vi "HFRR ADV v08 new software.vi"() -> ()   [LabVIEW 2025] (continued)
        n786 = case shown="True" "LIVE FEED MAX TEMP" {
          selector: "LIVE FEED MAX TEMP" -> [_ w1182]
          frame False {
          }
          frame True {
            n787 = Not(x=w1182) -> (.not. x?=w1181:bool)
            n788 = local write "LIVE FEED MAX TEMP"(w1181) -> ()
            n789 = call "CAMERA LIVE FEED FGV.vi"("Enum - Menu"=CAMERA_LIVE_FEED_ENUM."CAMERA RESTORE") -> ("error out"=w1172:errorcluster)  [unwired: 9 in, 1 out]
            n790 = Type Cast(type=30, x=0) -> (*(type *) &x=w1176:i32)
            n791 = Add(x=w1176, y=48) -> (x+y=w1177:i32)
            n792 = call "CAMERA LIVE FEED FGV.vi"("Enum - Menu"=CAMERA_LIVE_FEED_ENUM."CAMERA MODE SET", "error in (no error)"=w1172, "CAMERA MODE"=w1177) -> ("error out"=w1169:errorcluster)  [unwired: 7 in, 1 out]
            n793 = call "CAMERA LIVE FEED FGV.vi"("Enum - Menu"=CAMERA_LIVE_FEED_ENUM."CAMERA GRAY", "error in (no error)"=w1169) -> ("error out"=w1168:errorcluster)  [unwired: 8 in, 1 out]
            n794 = call "LIST FILE NAMES.vi"("error in (no error)"=w1168) -> ("error out"=w1178:errorcluster, "filenames"=w1179:string[])  [unwired: 9 in]
            n795 = property on="FILE 3" class="CmbBox"(error in=w1178, "Strings[]"=w1179) -> ()  [unwired: 1 in, 2 out]
          }
        }
        n796 = case shown="True" w1161 {
          selector: w1161 -> [_ w1167]
          frame False {
          }
          frame True {
            n797 = Not(x=w1167) -> (.not. x?=w1166:bool)
            n798 = local write "CAMERA ROI MIN TEMP"(w1166) -> ()
            n799 = call "IMAGE ANALYSIS.vi"("Enum"=POST_ANALYSIS_ENUM."MINIMIZE UI") -> ()  [unwired: 9 in, 2 out]
          }
        }
        n800 = local write "CAMERA ROI MAX TEMP"(TRUE ("CAMERA ROI MAX TEMP")) -> ()
        "LIVE FEED MIN TEMP" <- TRUE ("LIVE FEED MIN TEMP")
      }
      frame "Adv Scar Report" {
        n801 = local read "CAMERA ROI MAX TEMP"() -> (w1183:bool)
        n802 = local read "LIVE FEED MIN TEMP"() -> (w1185:bool)
        n803 = local write "LIVE FEED MAX TEMP"(TRUE ("LIVE FEED MAX TEMP")) -> ()
        n804 = case shown="True" w1185 {
          selector: w1185 -> [_ w1194]
          frame False {
          }
          frame True {
            n805 = Not(x=w1194) -> (.not. x?=w1193:bool)
            n806 = local write "LIVE FEED MIN TEMP"(w1193) -> ()
            n807 = call "CAMERA LIVE FEED FGV.vi"("Enum - Menu"=CAMERA_LIVE_FEED_ENUM."CAMERA MINIMIZE") -> ()  [unwired: 9 in, 2 out]
          }
        }
        n808 = case shown="True" w1183 {
          selector: w1183 -> [_ w1191]
          frame False {
          }
          frame True {
            n809 = Not(x=w1191) -> (.not. x?=w1189:bool)
            n810 = local write "CAMERA ROI MAX TEMP"(w1189) -> ()
            n811 = call "IMAGE ANALYSIS.vi"("Enum"=POST_ANALYSIS_ENUM."SHOW UI") -> ("error out"=w1188:errorcluster)  [unwired: 9 in, 1 out]
            n812 = call "LIST FILE NAMES.vi"("error in (no error)"=w1188) -> ("filenames"=w1187:string[])  [unwired: 9 in, 1 out]
            n813 = property on="Test File List :" class="CmbBox"("Strings[]"=w1187) -> ()  [unwired: 2 in, 2 out]
          }
        }
        n814 = local write "CAMERA ROI MIN TEMP"(TRUE ("CAMERA ROI MIN TEMP")) -> ()
      }
      frame "Compare Files" {
        n815 = local read "LIVE FEED MIN TEMP"() -> (w1197:bool)
        n816 = local write "LIVE FEED MAX TEMP"(TRUE ("LIVE FEED MAX TEMP")) -> ()
        n817 = local read "CAMERA ROI MIN TEMP"() -> (w1195:bool)
        n818 = case shown="True" w1197 {
          selector: w1197 -> [_ w1204]
          frame False {
          }
          frame True {
            n819 = Not(x=w1204) -> (.not. x?=w1203:bool)
            n820 = local write "LIVE FEED MIN TEMP"(w1203) -> ()
            n821 = call "CAMERA LIVE FEED FGV.vi"("Enum - Menu"=CAMERA_LIVE_FEED_ENUM."CAMERA MINIMIZE") -> ()  [unwired: 9 in, 2 out]
          }
        }
        n822 = case shown="True" w1195 {
          selector: w1195 -> [_ w1201]
          frame False {
          }
          frame True {
            n823 = Not(x=w1201) -> (.not. x?=w1200:bool)
            n824 = local write "CAMERA ROI MIN TEMP"(w1200) -> ()
            n825 = call "IMAGE ANALYSIS.vi"("Enum"=POST_ANALYSIS_ENUM."MINIMIZE UI") -> ()  [unwired: 9 in, 2 out]
          }
        }
        n826 = local write "CAMERA ROI MAX TEMP"(TRUE ("CAMERA ROI MAX TEMP")) -> ()
      }
      frame "About" {
        n827 = local read "LIVE FEED MIN TEMP"() -> (w1207:bool)
        n828 = local write "LIVE FEED MAX TEMP"(TRUE ("LIVE FEED MAX TEMP")) -> ()
        n829 = local read "CAMERA ROI MIN TEMP"() -> (w1206:bool)
        n830 = case shown="True" w1207 {
          selector: w1207 -> [_ w1214]
          frame False {
          }
          frame True {
            n831 = Not(x=w1214) -> (.not. x?=w1213:bool)
            n832 = local write "LIVE FEED MIN TEMP"(w1213) -> ()
            n833 = call "CAMERA LIVE FEED FGV.vi"("Enum - Menu"=CAMERA_LIVE_FEED_ENUM."CAMERA MINIMIZE") -> ()  [unwired: 9 in, 2 out]
          }
        }
        n834 = case shown="True" w1206 {
          selector: w1206 -> [_ w1211]
          frame False {
          }
          frame True {
            n835 = Not(x=w1211) -> (.not. x?=w1210:bool)
            n836 = local write "CAMERA ROI MIN TEMP"(w1210) -> ()
            n837 = call "IMAGE ANALYSIS.vi"("Enum"=POST_ANALYSIS_ENUM."MINIMIZE UI") -> ()  [unwired: 9 in, 2 out]
          }
        }
        n838 = local write "CAMERA ROI MAX TEMP"(TRUE ("CAMERA ROI MIN TEMP")) -> ()
      }
      frame "Advance" {
        n839 = local read "LIVE FEED MIN TEMP"() -> (w1217:bool)
        n840 = local write "LIVE FEED MAX TEMP"(TRUE ("LIVE FEED MAX TEMP")) -> ()
        n841 = local read "CAMERA ROI MIN TEMP"() -> (w1215:bool)
        n842 = case shown="True" w1217 {
          selector: w1217 -> [_ w1224]
          frame False {
          }
          frame True {
            n843 = Not(x=w1224) -> (.not. x?=w1223:bool)
            n844 = local write "LIVE FEED MIN TEMP"(w1223) -> ()
            n845 = call "CAMERA LIVE FEED FGV.vi"("Enum - Menu"=CAMERA_LIVE_FEED_ENUM."CAMERA MINIMIZE") -> ()  [unwired: 9 in, 2 out]
          }
        }
        n846 = local write "CAMERA ROI MAX TEMP"(TRUE ("CAMERA ROI MAX TEMP")) -> ()
        n847 = case shown="True" w1215 {
          selector: w1215 -> [_ w1221]
          frame False {
          }
          frame True {
            n848 = Not(x=w1221) -> (.not. x?=w1220:bool)
            n849 = local write "CAMERA ROI MIN TEMP"(w1220) -> ()
            n850 = call "IMAGE ANALYSIS.vi"("Enum"=POST_ANALYSIS_ENUM."MINIMIZE UI") -> ()  [unwired: 9 in, 2 out]
          }
        }
      }
      frame "Mooha" {
        n851 = local read "LIVE FEED MIN TEMP"() -> (w1227:bool)
        n852 = local write "LIVE FEED MAX TEMP"(TRUE ("LIVE FEED MAX TEMP")) -> ()
        n853 = local read "CAMERA ROI MIN TEMP"() -> (w1225:bool)
        n854 = case shown="True" w1227 {
          selector: w1227 -> [_ w1234]
          frame False {
          }
          frame True {
            n855 = Not(x=w1234) -> (.not. x?=w1233:bool)
            n856 = local write "LIVE FEED MIN TEMP"(w1233) -> ()
            n857 = call "CAMERA LIVE FEED FGV.vi"("Enum - Menu"=CAMERA_LIVE_FEED_ENUM."CAMERA MINIMIZE") -> ()  [unwired: 9 in, 2 out]
          }
        }
        n858 = local write "CAMERA ROI MAX TEMP"(TRUE ("CAMERA ROI MAX TEMP")) -> ()
        n859 = case shown="True" w1225 {
          selector: w1225 -> [_ w1231]
          frame False {
          }
          frame True {
            n860 = Not(x=w1231) -> (.not. x?=w1230:bool)
            n861 = local write "CAMERA ROI MIN TEMP"(w1230) -> ()
            n862 = call "IMAGE ANALYSIS.vi"("Enum"=POST_ANALYSIS_ENUM."MINIMIZE UI") -> ()  [unwired: 9 in, 2 out]
          }
        }
      }
    }
    n863 = local read "Auto Start Test"() -> (w971:bool)
    n864 = case shown="True" "sign in temp" {
      frame False {
      }
      frame True {
        w1007 = 1 ("y")
        n865 = local read "USERNAME"() -> (w1013:string)
        n866 = local read "USER ID"() -> (w1010:string)
        n867 = call <vilib>:"Trim Whitespace.vi"("string"=w1013) -> ("trimmed string"=w1012:string)  [unwired: 1 in]
        n868 = call <vilib>:"Trim Whitespace.vi"("string"=w1010) -> ("trimmed string"=w1011:string)  [unwired: 1 in]
        n869 = String Length(string=w1012) -> (length=w1009:i32)
        n870 = String Length(string=w1011) -> (length=w1008:i32)
        n871 = Greater?(x=w1009, y=w1007) -> (0:w1006:bool)
        n872 = Greater?(x=w1008, y=w1007) -> (0:w1005:bool)
        n873 = And(x=w1006, y=w1005) -> (x .and. y?=w1004:bool)
        n874 = case shown="True" w1004 {
          frame False {
            n875 = property on="Sign In" class="Bool (strict)"("DisabledEnum"=T16."Disabled" ("Disabled")) -> ()  [unwired: 2 in, 2 out]
          }
          frame True {
            n876 = property on="Sign In" class="Bool (strict)"("DisabledEnum"=T16."Enabled" ("Disabled")) -> ()  [unwired: 2 in, 2 out]
          }
        }
      }
    }
    n877 = local read "Air Temperature"() -> (w988:bool)
    n878 = local read "Coefficient Of Friction"() -> (w989:bool)
    n879 = case shown="False" w971 {
      frame False {
        n880 = local read "Auto stop temp"() -> (w1001:bool)
        n881 = case shown="True" w1001 {
          frame False {
          }
          frame True {
            n882 = local write "Auto Start Temp"(FALSE ("Auto Start Temp")) -> ()
          }
        }
      }
      frame True {
        "Auto stop temp" <- TRUE ("Auto stop temp")
      }
    }
    n883 = local read "Humidity"() -> (w987:bool)
    n884 = case shown="\"HOME\"" w998 {
      frame "HOME" {
        n885 = local write "main tab sub"(enum32{"Page 1", "Page 2"}."Page 1" ("main tab sub")) -> ()
      }
      frame Default {
        n886 = local write "main tab sub"(enum32{"Page 1", "Page 2"}."Page 2" ("main tab sub")) -> ()
      }
    }
    n887 = case shown="True" w997 {
      selector: w997 -> [_ w1340]
      frame False {
      }
      frame True {
        n888 = Not(x=w1340) -> (.not. x?=w1339:bool)
        n889 = local write "Sign In"(w1339) -> ()
        n890 = local write "Main Dashboard Buttons"(T22."Test Setup" ("Main Dashboard Buttons")) -> ()
      }
    }
    n891 = case shown="\"Numeric Display\", Default" "Num/Graph" {
      frame "Numeric Display", Default {
        n892 = property on="Single/Multiple" class="RadioBtnsControl (strict)"("Visible"=FALSE) -> ()  [unwired: 2 in, 2 out]
        n893 = property on="Single - Graph" class="Ring (strict)"("Visible"=FALSE) -> ()  [unwired: 2 in, 2 out]
        n894 = local write "Main Tab Display"(T4."Dashboard 1" ("Main Tab Display")) -> ()
      }
      frame "Graph Display" {
        n895 = property on="Single/Multiple" class="RadioBtnsControl (strict)"("Visible"=TRUE) -> ()  [unwired: 2 in, 2 out]
        n896 = case shown="\"Multiple\"" "Single/Multiple" {
          frame "Single ", Default {
            n897 = property on="Single - Graph" class="Ring (strict)"("Visible"=TRUE) -> ()  [unwired: 2 in, 2 out]
            n898 = local write "Main Tab Display"(T4."Dashboard 3" ("Main Tab Display")) -> ()
          }
          frame "Multiple" {
            n899 = property on="Single - Graph" class="Ring (strict)"("Visible"=FALSE) -> ()  [unwired: 2 in, 2 out]
            n900 = local write "Main Tab Display"(T4."Dashboard 2" ("Main Tab Display")) -> ()
          }
        }
      }
    }
    n901 = local read "Stroke"() -> (w986:bool)
    n902 = local read "USERNAME"() -> (w992:string)
    n903 = local read "USER ID"() -> (w991:string)
    n904 = case shown="True" w989 {
      selector: w989 -> [_ w1274]
      frame False {
      }
      frame True {
        n905 = Not(x=w1274) -> (.not. x?=w1273:bool)
        n906 = local write "Coefficient Of Friction"(w1273) -> ()
        n907 = local write "Tab Control 2"(T6."Coefficient Of Friction" ("Tab Control 2")) -> ()
      }
    }
    n908 = case shown="True" w988 {
      selector: w988 -> [_ w1271]
      frame False {
      }
      frame True {
        n909 = Not(x=w1271) -> (.not. x?=w1269:bool)
        n910 = local write "Air Temperature"(w1269) -> ()
        n911 = local write "Tab Control 2"(T6."Air Temperature" ("Tab Control 2")) -> ()
      }
    }
    n912 = local write "Operator ID"(w991) -> ()
    n913 = case shown="True" w986 {
      selector: w986 -> [_ w1265]
      frame False {
      }
      frame True {
        n914 = Not(x=w1265) -> (.not. x?=w1263:bool)
        n915 = local write "Stroke"(w1263) -> ()
        n916 = local write "Tab Control 2"(T6."Stroke" ("Tab Control 2")) -> ()
      }
    }
    n917 = local write "tested by"(w992) -> ()
    n918 = case shown="True" w987 {
      selector: w987 -> [_ w1268]
      frame False {
      }
      frame True {
        n919 = Not(x=w1268) -> (.not. x?=w1266:bool)
        n920 = local write "Humidity"(w1266) -> ()
        n921 = local write "Tab Control 2"(T6."Humidity" ("Tab Control 2")) -> ()
      }
    }
    n922 = case shown="\"Calibration\"" "Main Dashboard Buttons" {
      tunnel: [T2."HOME" ("Main Tab") T2."Test Setup" ("Main Tab") T2."Acquire" ("Main Tab") T2."Adv Scar" ("Main Tab") T2."Adv Scar Report" ("Main Tab") T2."Compare Files" ("Main Tab") T2."Calibration" ("Main Tab") T2."About" ("Main Tab") T2."Advance" ("Main Tab")] -> w970
      frame "Home", Default {
      }
      frame "Test Setup" {
      }
      frame "Dashboard" {
      }
      frame "Imaging" {
      }
      frame "Report" {
      }
      frame "Analysis" {
      }
      frame "Calibration" {
      }
      frame "About" {
      }
      frame "Advance" {
      }
    }
    n923 = Wait (ms)(milliseconds to wait=u32 100) -> ()  [unwired: 1 out]
    n924 = local read "Main Tab Display"() -> (w990:T4)
    n925 = local write "Main Tab"(w970) -> ()
    n926 = case shown="\"Dashboard 3\"" w990 {
      frame "Dashboard 1", Default {
        n927 = property on="Reset Graph" class="Bool (strict)"("Visible"=FALSE) -> ()  [unwired: 2 in, 2 out]
      }
      frame "Dashboard 2" {
        n928 = property on="Reset Graph" class="Bool (strict)"("Visible"=TRUE) -> ()  [unwired: 2 in, 2 out]
      }
      frame "Dashboard 3" {
        n929 = property on="Reset Graph" class="Bool (strict)"("Visible"=TRUE) -> ()  [unwired: 2 in, 2 out]
      }
    }
    n930 = local read "SCAR MEASURMENT"() -> (w978:enum32{"Auto Scar", "Manual Scar"})
    n931 = local read "Humidity"() -> (w993:bool)
    n932 = local read "Cap Live Image"() -> (w975:bool)
    n933 = local read "Sample Temperature"() -> (w985:bool)
    n934 = local read "Air Temp vs Humidity"() -> (w983:bool)
    n935 = local read "Frequency"() -> (w984:bool)
    n936 = case shown="False" w993 {
      frame False {
        n937 = local write "Humidity On Command"(TRUE ("Humidity On Command")) -> ()
        n938 = case shown="True" "Humidity Off Command" {
          selector: "Humidity Off Command" -> [_ w1281]
          frame False {
          }
          frame True {
            n939 = stacked-sequence {
              frame #0 {
                n940 = local read "WriteHumidity"() -> (w1283:string[])
                n941 = Insert Into Array(array=w1283, new element="R;1" ("new element/subarray")) -> (w1284:string[])  [unwired: 1 in]
                n942 = local write "WriteHumidity"(w1284) -> ()
              }
              frame #1 {
                n943 = Wait (ms)(milliseconds to wait=u32 2000) -> ()  [unwired: 1 out]
              }
              frame #2 {
                n944 = local read "EVENT LOG"() -> (w1290:string)
                n945 = local read "WriteHumidity"() -> (w1287:string[])
                n946 = call "Event Log.vi"("Content"="Humidity Control Off" ("string"), "EVENT LOG"=w1290) -> ("EVENT LOG"=w1291:string)  [unwired: 8 in, 1 out]
                n947 = local write "EVENT LOG"(w1291) -> ()
                n948 = Insert Into Array(array=w1287, new element="R;1" ("new element/subarray")) -> (w1288:string[])  [unwired: 1 in]
                n949 = local write "WriteHumidity"(w1288) -> ()
              }
            }
            n950 = Not(x=w1281) -> (.not. x?=w1280:bool)
            n951 = local write "Humidity Off Command"(w1280) -> ()
          }
        }
      }
      frame True {
        n952 = local write "Humidity Off Command"(TRUE ("Humidity Off Command")) -> ()
        n953 = case shown="False" "Humidity On Command" {
          selector: "Humidity On Command" -> [_ w1295]
          frame False {
          }
          frame True {
            n954 = stacked-sequence {
              frame #0 {
                n955 = local read "Set Rh"() -> (w1301:dbl)
                n956 = Number To Fractional String(number=w1301, precision (6)=i16 2) -> (F-format string=w1302:string)  [unwired: 2 in]
                n957 = local read "WriteHumidity"() -> (w1299:string[])
                n958 = Concatenate Strings("M;" ("new element/subarray"), w1302) -> (w1300:string)
                n959 = Insert Into Array(array=w1299, new element=w1300) -> (w1298:string[])  [unwired: 1 in]
                n960 = local write "WriteHumidity"(w1298) -> ()
              }
              frame #1 {
                n961 = Wait (ms)(milliseconds to wait=u32 1500) -> ()  [unwired: 1 out]
              }
              frame #2 {
                (unwired) "% RH" ("string")
                (unwired) i16 2 ("precision (6)")
                (unwired) "M;" ("new element/subarray")
                n962 = local read "Set Rh"() -> (w1309:dbl)
                n963 = Number To Fractional String(number=w1309, precision (6)=i16 2) -> (F-format string=w1306:string)  [unwired: 2 in]
                n964 = local read "WriteHumidity"() -> (w1311:string[])
                n965 = Concatenate Strings("M;" ("new element/subarray"), w1306) -> (w1310:string)
                n966 = Concatenate Strings("Humidity Set to : " ("string"), w1306, "% RH" ("string")) -> (w1304:string)
                n967 = Insert Into Array(array=w1311, new element=w1310) -> (w1312:string[])  [unwired: 1 in]
                n968 = disable-structure shown="Enabled" {
                  frame Enabled {
                    n969 = local read "EVENT LOG"() -> (w1315:string)
                    n970 = call "Event Log.vi"("Content"="Humidity Control On", "EVENT LOG"=w1315) -> ("EVENT LOG"=w1316:string)  [unwired: 8 in, 1 out]
                    n971 = local write "EVENT LOG"(w1316) -> ()
                  }
                  frame Disabled {
                  }
                }
                n972 = disable-structure shown="Enabled" {
                  disable-tunnel: w1304 -> [_ _]
                  frame Enabled {
                    n973 = local read "EVENT LOG"() -> (w1318:string)
                    n974 = call "Event Log.vi"("Content"="Humidity Control On", "EVENT LOG"=w1318) -> ("EVENT LOG"=w1319:string)  [unwired: 8 in, 1 out]
                    n975 = local write "EVENT LOG"(w1319) -> ()
                  }
                  frame Disabled {
                  }
                }
                n976 = local write "WriteHumidity"(w1312) -> ()
              }
            }
            n977 = Not(x=w1295) -> (.not. x?=w1294:bool)
            n978 = local write "Humidity On Command"(w1294) -> ()
          }
        }
      }
    }
    n979 = Equal?(x=w978, y=enum32{"Auto Scar", "Manual Scar"}."Auto Scar" ("SCAR MEASURMENT")) -> (x = y?=w974:bool)
    n980 = local read "TEST STANDARD"() -> (w981:T3)
    n981 = And(x=w975, y=w974) -> (x .and. y?=w976:bool)
    n982 = case shown="True" w976 {
      selector: w976 -> [_ w1080]
      tunnel: errorcluster {"status"=FALSE, "code"=0, "source"=""} ("error in (no error) 3") -> [_ w1081]
      frame False {
      }
      frame True {
        n983 = stacked-sequence {
          tunnel: w1081 -> [_ _ _ _ _ _ _ w1129]
          tunnel: w1080 -> [_ _ _ _ _ w1110 _ _]
          frame #0 {
            n984 = call "CAMERA LIVE FEED FGV.vi"("Enum - Menu"=CAMERA_LIVE_FEED_ENUM."CAMERA MINIMIZE") -> ()  [unwired: 9 in, 2 out]
          }
          frame #1 {
            n985 = property on="Auto Scar Check  2" class="Clust (strict)"("Visible"=TRUE) -> ()  [unwired: 2 in, 2 out]
          }
          frame #2 {
            n986 = String To Path(string="C:\\LAB-IQ\\Image Calibrate v01.dcf") -> (path=w1086:path)
            n987 = Open/Create/Replace File ("Open File")(file path (use dialog)=w1086) -> (refnum out=w1087:refnum<file>)  [unwired: 5 in, 2 out]
            n988 = for {
              N: 4 -> [_]
              tunnel: w1087 -> [w1093]
              i -> [w1089]
              n989 = Read from Text File ("Read File")(file (use dialog)=w1093) -> (text=w1094:string)  [unwired: 3 in, 3 out]
              n990 = String Subset(string=w1094, offset (0)=6, length (rest)=10 ("length (rest)")) -> (substring=w1090:string)
              n991 = Fract/Exp String To Number(string=w1090) -> (number=w1088:dbl)  [unwired: 3 in, 1 out]
              n992 = case shown="0" w1089 {
                tunnel: w1088 -> [w1095 w1096 _ w1097 _]
                frame 0 {
                  "5x Gain" <- w1095
                }
                frame 1 {
                  "10x Gain" <- w1096
                }
                frame 2 {
                }
                frame 3 {
                  "100x gain" <- w1097
                }
                frame 4, Default {
                }
              }
            }
          }
          frame #3 {
            n993 = local read "FILE 3"() -> (w1103:string)
            n994 = call <vilib>:"Trim Whitespace.vi"("string"="C:\\LAB-IQ\\images\\") -> ("trimmed string"=w1105:string)  [unwired: 1 in]
            n995 = String To Path(string=w1105) -> (path=w1104:path)
            n996 = Concatenate Strings(w1103, ".png" ("string")) -> (w1102:string)
            n997 = Build Path(base path=w1104, name or relative path=w1102) -> (appended path=w1100:path)
            "Image path" <- w1100
            n998 = Path To String(path=w1100) -> (string=w1099:string)
            n999 = call "CAMERA LIVE FEED FGV.vi"("Enum - Menu"=CAMERA_LIVE_FEED_ENUM."CAMERA SAVE", "Image Path"=w1099) -> ()  [unwired: 8 in, 2 out]
          }
          frame #4 {
            n1000 = One Button Dialog(message="Image saved successfully") -> ()  [unwired: 1 in, 1 out]
          }
          frame #5 {
            n1001 = local read "TEST STANDARD"() -> (w1109:T3)
            n1002 = local read "Magnification len live scar"() -> (w1121:string)
            n1003 = Not(x=w1110) -> (.not. x?=w1111:bool)
            n1004 = local write "Cap Live Image"(w1111) -> ()
            n1005 = case shown="\"ISO 12156\"" w1109 {
              tunnel: ["ASTM D6079" "ISO 12156"] -> w1108
              frame "ASTM D6079", Default {
              }
              frame "ISO 12156" {
              }
            }
            n1006 = case shown="\"5x\", Default" w1121 {
              tunnel: [w1124 w1125] -> w1120
              frame "5x", Default {
                n1007 = local read "5x Gain"() -> (w1124:dbl)
              }
              frame "10x" {
                # "5x"
                n1008 = local read "10x Gain"() -> (w1125:dbl)
              }
            }
            n1009 = local read "Image path"() -> (w1119:path)
            n1010 = local read "FILE 3"() -> (w1112:string)
            n1011 = call "EDGE DETCTION.vi"("GAIN VALUE"=w1120, "Image Path"=w1119) -> ("error out"=w1118:errorcluster, "return value"=w1117:cluster{string, string, dbl, dbl, dbl})  [unwired: 8 in]
            n1012 = Bundle By Name(cluster=T23 {"File Name"="", "Test Method"="", "Operator"="", "Fuel Description"="", "Date and time"=""} ("Main Ref"), "File Name"=w1112, "Test Method"=w1108) -> (w1113:T23)
            n1013 = call "duf file read.vi"("error in (no error)"=w1118, "Main Ref"=w1113) -> ("error out"=w1116:errorcluster, "Main Ref 2"=w1114:T23)  [unwired: 8 in]
            n1014 = call "EDGE DETECTION REPORT.vi"("error in (no error)"=w1116, "return value 2"=w1117, "Main Ref"=w1114) -> ()  [unwired: 8 in, 1 out]
          }
          frame #6 {
            n1015 = property on="Auto Scar Check  2" class="Clust (strict)"("Visible"=FALSE) -> ()  [unwired: 2 in, 2 out]
          }
          frame #7 {
            n1016 = call "CAMERA LIVE FEED FGV.vi"("Enum - Menu"=CAMERA_LIVE_FEED_ENUM."CAMERA MINIMIZE", "error in (no error)"=w1129) -> ()  [unwired: 8 in, 2 out]
            n1017 = local write "Main Dashboard Buttons"(T1."Home" ("Main Dashboard Buttons")) -> ()
            n1018 = local write "Main Tab"(T2."HOME" ("Main Tab")) -> ()
          }
        }
      }
    }
    n1019 = local read "Heater Button"() -> (w982:bool)
    n1020 = case shown="True" w984 {
      selector: w984 -> [_ w1259]
      frame False {
      }
      frame True {
        n1021 = Not(x=w1259) -> (.not. x?=w1257:bool)
        n1022 = local write "Frequency"(w1257) -> ()
        n1023 = local write "Tab Control 2"(T6."Frequency" ("Tab Control 2")) -> ()
      }
    }
    n1024 = case shown="True" w983 {
      selector: w983 -> [_ w1256]
      frame False {
      }
      frame True {
        n1025 = Not(x=w1256) -> (.not. x?=w1254:bool)
        n1026 = local write "Air Temp vs Humidity"(w1254) -> ()
        n1027 = local write "Tab Control 2"(T6."Air Temp vs Rh" ("Tab Control 2")) -> ()
      }
    }
    n1028 = case shown="True" w985 {
      selector: w985 -> [_ w1262]
      frame False {
      }
      frame True {
        n1029 = Not(x=w1262) -> (.not. x?=w1260:bool)
        n1030 = local write "Sample Temperature"(w1260) -> ()
        n1031 = local write "Tab Control 2"(T6."Sample Temperature" ("Tab Control 2")) -> ()
      }
    }
    n1032 = case shown="\"Custom\"" w981 {
      frame "ASTM D6079", Default {
        w1235 = "ASTM D6079 TEST CONDITIONS" ("Standard 2")
        n1033 = local write "Standard 2"(w1235) -> ()
        n1034 = local write "Standard"(w1235) -> ()
      }
      frame "ISO 12156" {
        w1236 = "ISO 12156 TEST CONDITIONS" ("Standard 2")
        n1035 = local write "Standard 2"(w1236) -> ()
        n1036 = local write "Standard"(w1236) -> ()
      }
      frame "CEC F-096-A-06" {
        w1237 = "CEC F-096-A-06 TEST CONDITIONS" ("Standard 2")
        n1037 = local write "Standard 2"(w1237) -> ()
        n1038 = local write "Standard"(w1237) -> ()
      }
      frame "Custom" {
        w1238 = "CUSTOM TEST CONDITIONS" ("Standard 2")
        n1039 = local write "Standard 2"(w1238) -> ()
        n1040 = local write "Standard"(w1238) -> ()
      }
    }
    n1041 = case shown="True" w982 {
      frame False {
        n1042 = local write "Temperature On Command"(TRUE ("Temperature On Command")) -> ()
        n1043 = case shown="True" "Temperature Off Command" {
          selector: "Temperature Off Command" -> [_ w1242]
          frame False {
          }
          frame True {
            n1044 = Not(x=w1242) -> (.not. x?=w1241:bool)
            n1045 = local read "EVENT LOG"() -> (w1245:string)
            n1046 = local write "Temperature Off Command"(w1241) -> ()
            n1047 = call "Event Log.vi"("Content"="Heater Off", "EVENT LOG"=w1245) -> ("EVENT LOG"=w1244:string)  [unwired: 8 in, 1 out]
            n1048 = local write "EVENT LOG"(w1244) -> ()
          }
        }
      }
      frame True {
        n1049 = local write "Temperature Off Command"(TRUE ("Temperature Off Command")) -> ()
        n1050 = case shown="True" "Temperature On Command" {
          selector: "Temperature On Command" -> [_ w1249]
          frame False {
          }
          frame True {
            n1051 = Not(x=w1249) -> (.not. x?=w1248:bool)
            n1052 = local write "Temperature On Command"(w1248) -> ()
            n1053 = disable-structure shown="Enabled" {
              disable-tunnel: "Heater On" -> [w1251 _]
              frame Enabled {
                n1054 = local read "EVENT LOG"() -> (w1252:string)
                n1055 = call "Event Log.vi"("Content"=w1251, "EVENT LOG"=w1252) -> ("EVENT LOG"=w1253:string)  [unwired: 8 in, 1 out]
                n1056 = local write "EVENT LOG"(w1253) -> ()
              }
              frame Disabled {
              }
            }
          }
        }
      }
    }
    n1057 = local read "Main Tab"() -> (w973:T2)
    n1058 = case shown="\"About\"" w973 {
      frame "HOME", Default {
        w1016 = T16."Enabled" ("Disabled")
        n1059 = local read "Service Password enable"() -> (w1018:bool)
        n1060 = property on="Imaging" class="Bool (strict)"("DisabledEnum"=w1016) -> ()  [unwired: 2 in, 2 out]
        n1061 = property on="Dashboard" class="Bool (strict)"("DisabledEnum"=w1016) -> ()  [unwired: 2 in, 2 out]
        n1062 = property on="Test Setup" class="Bool (strict)"("DisabledEnum"=w1016) -> ()  [unwired: 2 in, 2 out]
        n1063 = property on="Analysis" class="Bool (strict)"("DisabledEnum"=w1016) -> ()  [unwired: 2 in, 2 out]
        n1064 = property on="Home" class="Bool (strict)"("DisabledEnum"=w1016) -> ()  [unwired: 2 in, 2 out]
        n1065 = property on="Report" class="Bool (strict)"("DisabledEnum"=w1016) -> ()  [unwired: 2 in, 2 out]
        n1066 = property on="Main Dashboard Buttons" class="RadioBtnsControl (strict)"("DisabledEnum"=w1016) -> ()  [unwired: 2 in, 2 out]
        n1067 = property on="Calibration" class="Bool (strict)"("DisabledEnum"=w1016) -> ()  [unwired: 2 in, 2 out]
        n1068 = case shown="True" w1018 {
          tunnel: [T16."Disabled" ("Disabled") T16."Enabled" ("Disabled")] -> w1017
          frame False {
          }
          frame True {
          }
        }
        n1069 = property on="About" class="Bool (strict)"("DisabledEnum"=w1017) -> ()  [unwired: 2 in, 2 out]
      }
      frame "Test Setup" {
        w1023 = T16."Enabled" ("Disabled")
        n1070 = local read "Service Password enable"() -> (w1022:bool)
        n1071 = property on="Dashboard" class="Bool (strict)"("DisabledEnum"=T16."Disabled" ("Disabled")) -> ()  [unwired: 2 in, 2 out]
        n1072 = property on="Imaging" class="Bool (strict)"("DisabledEnum"=w1023) -> ()  [unwired: 2 in, 2 out]
        n1073 = property on="Analysis" class="Bool (strict)"("DisabledEnum"=w1023) -> ()  [unwired: 2 in, 2 out]
        n1074 = property on="Home" class="Bool (strict)"("DisabledEnum"=w1023) -> ()  [unwired: 2 in, 2 out]
        n1075 = property on="Report" class="Bool (strict)"("DisabledEnum"=w1023) -> ()  [unwired: 2 in, 2 out]
        n1076 = property on="Test Setup" class="Bool (strict)"("DisabledEnum"=w1023) -> ()  [unwired: 2 in, 2 out]
        n1077 = case shown="True" w1022 {
          tunnel: [T16."Disabled" ("Disabled") T16."Enabled" ("Disabled")] -> w1021
          frame False {
          }
          frame True {
          }
        }
        n1078 = property on="About" class="Bool (strict)"("DisabledEnum"=w1021) -> ()  [unwired: 2 in, 2 out]
      }
      frame "Adv Scar" {
        w1030 = T16."Enabled" ("Disabled")
        n1079 = property on="Dashboard" class="Bool (strict)"("DisabledEnum"=T16."Disabled" ("Disabled")) -> ()  [unwired: 2 in, 2 out]
        n1080 = property on="Imaging" class="Bool (strict)"("DisabledEnum"=w1030) -> ()  [unwired: 2 in, 2 out]
        n1081 = property on="Analysis" class="Bool (strict)"("DisabledEnum"=w1030) -> ()  [unwired: 2 in, 2 out]
        n1082 = property on="Home" class="Bool (strict)"("DisabledEnum"=w1030) -> ()  [unwired: 2 in, 2 out]
        n1083 = property on="Report" class="Bool (strict)"("DisabledEnum"=w1030) -> ()  [unwired: 2 in, 2 out]
        n1084 = property on="Test Setup" class="Bool (strict)"("DisabledEnum"=w1030) -> ()  [unwired: 2 in, 2 out]
        n1085 = local read "Service Password enable"() -> (w1028:bool)
        n1086 = case shown="True" w1028 {
          tunnel: [T16."Disabled" ("Disabled") T16."Enabled" ("Disabled")] -> w1027
          frame False {
          }
          frame True {
          }
        }
        n1087 = property on="About" class="Bool (strict)"("DisabledEnum"=w1027) -> ()  [unwired: 2 in, 2 out]
      }
      frame "Calibration" {
        w1033 = T16."Enabled" ("Disabled")
        n1088 = property on="Dashboard" class="Bool (strict)"("DisabledEnum"=T16."Disabled" ("Disabled")) -> ()  [unwired: 2 in, 2 out]
        n1089 = property on="Imaging" class="Bool (strict)"("DisabledEnum"=w1033) -> ()  [unwired: 2 in, 2 out]
        n1090 = property on="Analysis" class="Bool (strict)"("DisabledEnum"=w1033) -> ()  [unwired: 2 in, 2 out]
        n1091 = property on="Home" class="Bool (strict)"("DisabledEnum"=w1033) -> ()  [unwired: 2 in, 2 out]
        n1092 = property on="Report" class="Bool (strict)"("DisabledEnum"=w1033) -> ()  [unwired: 2 in, 2 out]
        n1093 = property on="Test Setup" class="Bool (strict)"("DisabledEnum"=w1033) -> ()  [unwired: 2 in, 2 out]
        n1094 = local read "Service Password enable"() -> (w1035:bool)
        n1095 = property on="Calibration" class="Bool (strict)"("DisabledEnum"=w1033) -> ()  [unwired: 2 in, 2 out]
        n1096 = case shown="True" w1035 {
          tunnel: [T16."Disabled" ("Disabled") T16."Enabled" ("Disabled")] -> w1034
          frame False {
          }
          frame True {
          }
        }
        n1097 = property on="About" class="Bool (strict)"("DisabledEnum"=w1034) -> ()  [unwired: 2 in, 2 out]
      }
      frame "Adv Scar Report" {
        w1041 = T16."Enabled" ("Disabled")
        n1098 = property on="Dashboard" class="Bool (strict)"("DisabledEnum"=T16."Disabled" ("Disabled")) -> ()  [unwired: 2 in, 2 out]
        n1099 = property on="Imaging" class="Bool (strict)"("DisabledEnum"=w1041) -> ()  [unwired: 2 in, 2 out]
        n1100 = property on="Analysis" class="Bool (strict)"("DisabledEnum"=w1041) -> ()  [unwired: 2 in, 2 out]
        n1101 = property on="Home" class="Bool (strict)"("DisabledEnum"=w1041) -> ()  [unwired: 2 in, 2 out]
        n1102 = property on="Report" class="Bool (strict)"("DisabledEnum"=w1041) -> ()  [unwired: 2 in, 2 out]
        n1103 = property on="Test Setup" class="Bool (strict)"("DisabledEnum"=w1041) -> ()  [unwired: 2 in, 2 out]
        n1104 = local read "Service Password enable"() -> (w1040:bool)
        n1105 = case shown="True" w1040 {
          tunnel: [T16."Disabled" ("Disabled") T16."Enabled" ("Disabled")] -> w1039
          frame False {
          }
          frame True {
          }
        }
        n1106 = property on="About" class="Bool (strict)"("DisabledEnum"=w1039) -> ()  [unwired: 2 in, 2 out]
      }
      frame "Compare Files" {
        w1047 = T16."Enabled" ("Disabled")
        n1107 = local read "Service Password enable"() -> (w1046:bool)
        n1108 = property on="Dashboard" class="Bool (strict)"("DisabledEnum"=T16."Disabled" ("Disabled")) -> ()  [unwired: 2 in, 2 out]
        n1109 = property on="Imaging" class="Bool (strict)"("DisabledEnum"=w1047) -> ()  [unwired: 2 in, 2 out]
        n1110 = property on="Analysis" class="Bool (strict)"("DisabledEnum"=w1047) -> ()  [unwired: 2 in, 2 out]
        n1111 = property on="Home" class="Bool (strict)"("DisabledEnum"=w1047) -> ()  [unwired: 2 in, 2 out]
        n1112 = property on="Report" class="Bool (strict)"("DisabledEnum"=w1047) -> ()  [unwired: 2 in, 2 out]
        n1113 = property on="Test Setup" class="Bool (strict)"("DisabledEnum"=w1047) -> ()  [unwired: 2 in, 2 out]
        n1114 = case shown="True" w1046 {
          tunnel: [T16."Disabled" ("Disabled") T16."Enabled" ("Disabled")] -> w1045
          frame False {
          }
          frame True {
          }
        }
        n1115 = property on="About" class="Bool (strict)"("DisabledEnum"=w1045) -> ()  [unwired: 2 in, 2 out]
      }
      frame "Acquire" {
        n1116 = local read "Service Password enable"() -> (w1052:bool)
        n1117 = property on="Test Setup" class="Bool (strict)"("DisabledEnum"=T16."Disabled" ("Disabled")) -> ()  [unwired: 2 in, 2 out]
        n1118 = local read "Auto Start Test"() -> (w1054:bool)
        n1119 = local read "RUN"() -> (w1056:bool)
        n1120 = case shown="True" w1052 {
          tunnel: [T16."Disabled" ("Disabled") T16."Enabled" ("Disabled")] -> w1053
          frame False {
          }
          frame True {
          }
        }
        n1121 = Or(x=w1056, y=w1054) -> (x .or. y?=w1055:bool)
        n1122 = case shown="True" w1055 {
          tunnel: [T16."Enabled" ("Disabled") T16."Disabled" ("Disabled")] -> w1051
          frame False {
          }
          frame True {
          }
        }
        n1123 = property on="About" class="Bool (strict)"("DisabledEnum"=w1053) -> ()  [unwired: 2 in, 2 out]
        n1124 = property on="Imaging" class="Bool (strict)"("DisabledEnum"=w1051) -> ()  [unwired: 2 in, 2 out]
        n1125 = property on="Dashboard" class="Bool (strict)"("DisabledEnum"=w1051) -> ()  [unwired: 2 in, 2 out]
        n1126 = property on="Analysis" class="Bool (strict)"("DisabledEnum"=w1051) -> ()  [unwired: 2 in, 2 out]
        n1127 = property on="Home" class="Bool (strict)"("DisabledEnum"=w1051) -> ()  [unwired: 2 in, 2 out]
        n1128 = property on="Report" class="Bool (strict)"("DisabledEnum"=w1051) -> ()  [unwired: 2 in, 2 out]
        n1129 = property on="Calibration" class="Bool (strict)"("DisabledEnum"=w1051) -> ()  [unwired: 2 in, 2 out]
      }
      frame "About" {
        n1130 = local read "FILE"() -> (w1070:string)
        n1131 = local read "TEST FILE NAM,E SAVED"() -> (w1063:bool)
        n1132 = call <vilib>:"Trim Whitespace.vi"("string"=w1070) -> ("trimmed string"=w1069:string)  [unwired: 1 in]
        n1133 = local read "Auto Start Test"() -> (w1073:bool)
        n1134 = String Length(string=w1069) -> (length=w1068:i32)
        n1135 = Greater?(x=w1068, y=1) -> (0:w1065:bool)
        n1136 = And(x=w1065, y=w1063) -> (x .and. y?=w1064:bool)
        n1137 = local read "RUN"() -> (w1075:bool)
        n1138 = case shown="True" w1064 {
          tunnel: [T16."Disabled" ("Disabled") T16."Enabled" ("Disabled")] -> w1066
          frame False {
          }
          frame True {
          }
        }
        n1139 = Or(x=w1075, y=w1073) -> (x .or. y?=w1074:bool)
        n1140 = property on="About" class="Bool (strict)"("DisabledEnum"=T16."Enabled" ("Disabled")) -> ()  [unwired: 2 in, 2 out]
        n1141 = case shown="False" w1074 {
          tunnel: [T16."Enabled" ("Disabled") T16."Disabled" ("Disabled")] -> w1072
          frame False {
          }
          frame True {
          }
        }
        n1142 = property on="Dashboard" class="Bool (strict)"("DisabledEnum"=w1066) -> ()  [unwired: 2 in, 2 out]
        n1143 = property on="Test Setup" class="Bool (strict)"("DisabledEnum"=T16."Disabled" ("Disabled")) -> ()  [unwired: 2 in, 2 out]
        n1144 = property on="Imaging" class="Bool (strict)"("DisabledEnum"=w1072) -> ()  [unwired: 2 in, 2 out]
        n1145 = property on="Analysis" class="Bool (strict)"("DisabledEnum"=w1072) -> ()  [unwired: 2 in, 2 out]
        n1146 = property on="Home" class="Bool (strict)"("DisabledEnum"=w1072) -> ()  [unwired: 2 in, 2 out]
        n1147 = property on="Report" class="Bool (strict)"("DisabledEnum"=w1072) -> ()  [unwired: 2 in, 2 out]
      }
    }
    n1148 = local read "Quit"() -> (w1000:bool)
    "Single" <- "Single - Graph"
  }
  n1149 = disable-structure shown="Disabled" {
    disable-tunnel: [w1344 _] -> w39
    disable-tunnel: _ -> [w1343 _]
    frame Disabled {
      n1150 = while {
        tunnel: w1343 -> [_]
        tunnel: [w1345] -> w1344
        tunnel: [w1346] -> _
        i -> [w1346]
        stop <- w1345 stop-if-true
        w1362 = u16 10 items=["1.0"=10, "1.5"=15, "2.0"=20] ("stop bits (10: 1 bit)")
        n1151 = Wait (ms)(milliseconds to wait=u32 10) -> ()  [unwired: 1 out]
        n1152 = call-poly "VISA Configure Serial Port"("VISA resource name"=refnum<visa-resource-name> "ASRL1::INSTR" ("COM PORT"), "timeout (10sec)"=u32 10, "baud rate (9600)"=u32 57600, "data bits (8)"=u16 8, "stop bits (10: 1 bit)"=w1362) -> ("VISA resource name out"=w1348:refnum<visa-resource-name>, "error out"=w1357:errorcluster)  [unwired: 9 in]
        n1153 = VISA Read(VISA resource name=w1348, byte count=u32 2 ("byte count (0)")) -> (read buffer=w1356:string)  [unwired: 1 in, 3 out]
        n1154 = String Subset(string=w1356, offset (0)=0, length (rest)=2 ("length (rest)")) -> (substring=w1355:string)
        n1155 = Match Pattern(string=w1355, regular expression="<>") -> (offset past match=w1352:i32)  [unwired: 1 in, 3 out]
        n1156 = Greater Or Equal?(x=w1352, y=0) -> (x >= y?=w1347:bool)
        n1157 = case shown="True" w1347 {
          tunnel: w1348 -> [_ w1366]
          tunnel: w1357 -> [_ w1365]
          frame False {
          }
          frame True {
            n1158 = VISA Read(VISA resource name=w1366, byte count=u32 32 ("byte count (0)"), error in (no error)=w1365) -> (read buffer=w1364:string)  [unwired: 3 out]
            n1159 = String Subset(string=w1364, offset (0)=0, length (rest)=8 ("length (rest)")) -> (substring=w1368:string)
            n1160 = String Subset(string=w1364, offset (0)=8, length (rest)=8 ("length (rest)")) -> (substring=w1369:string)
            n1161 = Decimal String To Number(string=w1369) -> (number=w1376:i32)  [unwired: 2 in, 1 out]
            n1162 = Decimal String To Number(string=w1368) -> (number=w1372:i32)  [unwired: 2 in, 1 out]
            n1163 = Divide(x=w1376, y=10000) -> ()  [unwired: 1 out]
            n1164 = Divide(x=w1372, y=1000000) -> ()  [unwired: 1 out]
          }
        }
        n1165 = local read "Quit"() -> (w1345:bool)
      }
    }
    frame Enabled {
    }
  }
  n1166 = while {
    shift-right: [w1391] -> w52
    shift-left: _ -> [w1382]
    shift-right: [w1390] -> w51
    shift-left: errorcluster {"status"=TRUE, "code"=0, "source"="Init"} ("error IO") -> [w1384]
    tunnel: [w1379] -> w42
    tunnel: [w1389] -> _
    i -> [w1389]
    stop <- w1379 stop-if-true
    n1167 = local read "Port 1a"() -> (w1385:bool)
    n1168 = local read "Port 3"() -> (w1386:bool)
    n1169 = local read "Com Port 1"() -> (w1383:refnum<visa-resource-name>)
    n1170 = Or(x=w1386, y=w1385) -> (x .or. y?=w1388:bool)
    n1171 = Unbundle(w1384) -> ("status"=→"Port 3":bool)  [unwired: 2 out]
    n1172 = Not Equal?(x=w1383, y=w1382) -> (x != y?=w1380:bool)
    n1173 = case shown="True" w1388 {
      frame False {
        w1394 = TRUE ("Visible")
        n1174 = property on="Port 1a" class="Bool (strict)"("Visible"=w1394) -> ()  [unwired: 2 in, 2 out]
        n1175 = property on="Port 3" class="Bool (strict)"("Visible"=w1394) -> ()  [unwired: 2 in, 2 out]
      }
      frame True {
        w1395 = TRUE ("Visible")
        n1176 = property on="Port 1a" class="Bool (strict)"("Visible"=w1395) -> ()  [unwired: 2 in, 2 out]
        n1177 = property on="Port 3" class="Bool (strict)"("Visible"=w1395) -> ()  [unwired: 2 in, 2 out]
      }
    }
    n1178 = Wait (ms)(milliseconds to wait=u32 40) -> ()  [unwired: 1 out]
    n1179 = case shown="True" w1380 {
      tunnel: [w1392 errorcluster {"status"=TRUE, "code"=0, "source"="Init"} ("error out")] -> w1381
      tunnel: w1384 -> [w1392 _]
      frame False {
      }
      frame True {
      }
    }
    n1180 = case shown="Error" w1381 {
      selector: w1381 -> [w1403 w1430]
      tunnel: [w1397 w1434] -> w1391
      tunnel: [w1405 w1428] -> w1390
      tunnel: w1382 -> [w1404 w1432]
      frame No Error {
        n1181 = property class="Instr"(reference=w1404, error in=w1403) -> (reference out=w1401:refnum<visa-resource-name>, error out=w1402:errorcluster, "Serial Settings:Number of Bytes at Serial Port"=w1398:u32)
        n1182 = Greater?(x=w1398, y=u32 5) -> (0:w1396:bool)
        n1183 = Not(x=w1396) -> (.not. x?=→"Port 1a":bool)
        n1184 = while {
          tunnel: [w1423] -> w1405
          tunnel: [w1422] -> w1406
          tunnel: w1402 -> [w1421]
          tunnel: w1401 -> [w1420]
          stop <- TRUE stop-if-true
          n1185 = property class="Instr" props=["Serial Settings:Number of Bytes at Serial Port"](reference=w1420, error in=w1421) -> (reference out=w1425:refnum<visa-resource-name>, error out=w1424:errorcluster)  [unwired: 1 out]
          n1186 = VISA Read(VISA resource name=w1425, byte count=u32 50, error in (no error)=w1424) -> (VISA resource name out=w1422:refnum<visa-resource-name>, read buffer=w1407:string, error out=w1423:errorcluster)  [unwired: 1 out]
          "UNI READ" <- w1407
          n1187 = Spreadsheet String To Array(delimiter (Tab)=";", format string="", spreadsheet string=w1407, array type (2D Dbl)=dbl[] []) -> (array=w1417:dbl[])
          n1188 = Index Array(array=w1417) -> (element #1=→"LVDT MIN":dbl, element #2=→"LVDT MAX":dbl, element #3=→"LVDT Peak":dbl, element #4=→"pizo raw":dbl, element #5=→"Friction":dbl, element #6=→"cof 2":dbl)  [unwired: 6 in]
        }
        n1189 = VISA Flush I/O Buffer(VISA resource name=w1406) -> (VISA resource name out=w1397:refnum<visa-resource-name>)  [unwired: 2 in, 1 out]
      }
      frame Error {
        w1440 = u16 0 items=["None", "XON/XOFF", "RTS/CTS", "XON/XOFF & RTS/CTS", "DTR/DSR", "XON/XOFF & DTR/DSR"] ("flow control (0:none)  2")
        w1438 = u16 10 items=["1.0"=10, "1.5"=15, "2.0"=20] ("stop bits 2")
        w1436 = u16 0 items=["None", "Odd", "Even", "Mark", "Space"] ("parity 2")
        w1437 = u32 10000  # timeout (10sec)
        n1190 = VISA Close(VISA resource name=w1432, error in (no error)=w1430) -> (error out=w1433:errorcluster)
        n1191 = local write "Port 1a"(FALSE ("Port 1a")) -> ()
        n1192 = local read "Com Port 1"() -> (w1427:refnum<visa-resource-name>)
        n1193 = call <vilib>:"Clear Errors.vi"("error in (no error)"=w1433) -> ("error out"=w1431:errorcluster)  [unwired: 5 in, 1 out]
        n1194 = call-poly "VISA Configure Serial Port"("VISA resource name"=w1427, "timeout (10sec)"=w1437, "baud rate (9600)"=u32 250000 ("baud rate  2"), "data bits (8)"=u16 8 ("data bits  2"), "parity (0:none)"=w1436, "error in (no error)"=w1431, "stop bits (10: 1 bit)"=w1438, "flow control (0:none)"=w1440) -> ("VISA resource name out"=w1441:refnum<visa-resource-name>, "error out"=w1442:errorcluster)  [unwired: 6 in]
        n1195 = flat-sequence {
          tunnel: w1441 -> [w1444]
          tunnel: w1442 -> [w1443]
          tunnel: [w1444] -> w1434
          tunnel: [w1443] -> w1428
          frame #0 {
            n1196 = Wait (ms)(milliseconds to wait=u32 50) -> ()  [unwired: 1 out]
          }
        }
        "Residual Uno" <- ""
        "Port 1 Error" <- w1428
      }
    }
    n1197 = local read "Quit"() -> (w1379:bool)
    "Error Uno" <- w1384
  }
  n1198 = while {
    stop <- w1451 stop-if-true
    # "V0OLTAGE TO STROKE (peice vise calibration)"
    n1199 = Wait (ms)(milliseconds to wait=u32 10) -> ()  [unwired: 1 out]
    n1200 = local read "LVDT Peak"() -> (w1448:dbl)
    n1201 = formula code="// Dynamic Parameterized Linear Interpolation Node\n// Inputs: vpp_val, voltages (Array), distances (Array)\n// Outputs: stroke\n\nint i = 0;\nint segments = 11; // 12 points make 11 interpolation segments\n\n// 1. Lower Boundary Clamp\nif (vpp_val <= voltages[0]) {\n    stroke = distances[0];\n}\n// 2. Upper Boundary Clamp\nelse if (vpp_val >= voltages[segments]) {\n    stroke = distances[segments];\n}\n// 3. Dynamic Segment Search Loop\nelse {\n    stroke = distances[0]; // Fallback baseline\n    for (i = 0; i < segments; i++) {\n        if (vpp_val >= voltages[i] && vpp_val <= voltages[i+1]) {\n            // Standard linear interpolation formula using array lookups\n            stroke = distances[i] + (vpp_val - voltages[i]) * (distances[i+1] - distances[i]) / (voltages[i+1] - voltages[i]);\n            break; // Segment found, safely exit the loop\n        }\n    }\n}"("vpp_val"=w1448, "voltages"="calibration values", "distances"="STROKE") -> ("stroke"=→"LVDT STROKE":dbl)
    n1202 = local read "Quit"() -> (w1451:bool)
  }
  n1203 = while {
    stop <- w1471 stop-if-true
    n1204 = call <vilib>:"High Resolution Polling Wait.vi"("seconds to wait"=0.02) -> ()  [unwired: 10 in, 1 out]
    n1205 = local read "Due read"() -> (w1469:string)
    n1206 = Spreadsheet String To Array(delimiter (Tab)=";", format string="", spreadsheet string=w1469, array type (2D Dbl)=string[] []) -> (array=w1466:string[])
    n1207 = Fract/Exp String To Number(string=w1466) -> (number=w1465:dbl[])  [unwired: 3 in, 1 out]
    n1208 = Index Array(array=w1465) -> (element #1=→"Sample Temperature":dbl, element #2=→"Target Sample Temperature":dbl, element #3=→"Current Duty Cycle":dbl, element #4=→"Ambient Temperature":dbl, element #5=→"Dac Status":dbl, element #6=→"Vpp":dbl, element #7=→"Active Error Code":dbl, element #8=→"Kp":dbl, element #9=→"Ki":dbl, element #10=→"Kd":dbl, element #11=→"SampleRaw":dbl, element #12=→"AmbRaw":dbl)  [unwired: 12 in]
    n1209 = local read "Quit"() -> (w1471:bool)
  }
  n1210 = while {
    shift-right: [w1485] -> w37
    shift-left: _ -> [w1476]
    shift-right: [w1484] -> w36
    shift-left: errorcluster {"status"=FALSE, "code"=0, "source"="Init"} ("error out") -> [w1478]
    tunnel: [w1473] -> w41
    tunnel: [w1483] -> _
    i -> [w1483]
    stop <- w1473 stop-if-true
    n1211 = local read "Com Port 2"() -> (w1477:refnum<visa-resource-name>)
    n1212 = local read "Port 2a"() -> (w1479:bool)
    n1213 = Unbundle(w1478) -> ("status"=→"Port 4":bool)  [unwired: 2 out]
    n1214 = call <vilib>:"High Resolution Polling Wait.vi"("seconds to wait"=0.02) -> ()  [unwired: 10 in, 1 out]
    n1215 = local read "Port 4"() -> (w1480:bool)
    n1216 = Not Equal?(x=w1477, y=w1476) -> (x != y?=w1475:bool)
    n1217 = Or(x=w1480, y=w1479) -> (x .or. y?=w1482:bool)
    n1218 = case shown="False" w1482 {
      frame False {
        w1488 = TRUE ("Visible")
        n1219 = property on="Port 2a" class="Bool (strict)"("Visible"=w1488) -> ()  [unwired: 2 in, 2 out]
        n1220 = property on="Port 4" class="Bool (strict)"("Visible"=w1488) -> ()  [unwired: 2 in, 2 out]
      }
      frame True {
        w1489 = TRUE ("Visible")
        n1221 = property on="Port 2a" class="Bool (strict)"("Visible"=w1489) -> ()  [unwired: 2 in, 2 out]
        n1222 = property on="Port 4" class="Bool (strict)"("Visible"=w1489) -> ()  [unwired: 2 in, 2 out]
      }
    }
    n1223 = case shown="True" w1475 {
      tunnel: [w1486 errorcluster {"status"=TRUE, "code"=0, "source"="Init"} ("error out")] -> w1474
      tunnel: w1478 -> [w1486 _]
      frame False {
      }
      frame True {
      }
    }
    n1224 = case shown="No Error" w1474 {
      selector: w1474 -> [w1500 w1531]
      tunnel: [w1493 w1536] -> w1485
      tunnel: [w1501 w1529] -> w1484
      tunnel: w1476 -> [w1503 w1534]
      frame No Error {
        n1225 = property class="Instr" props=["Serial Settings:Number of Bytes at Serial Port"](reference=w1503, error in=w1500) -> (reference out=w1494:refnum<visa-resource-name>, error out=w1499:errorcluster)  [unwired: 1 out]
        n1226 = while {
          tunnel: [w1511] -> w1495
          tunnel: [w1510] -> w1496
          tunnel: w1499 -> [w1509]
          tunnel: w1494 -> [w1508]
          tunnel: [w1507] -> _
          i -> [w1507]
          stop <- TRUE stop-if-true
          n1227 = property class="Instr" props=["Serial Settings:Number of Bytes at Serial Port"](reference=w1508, error in=w1509) -> (reference out=w1513:refnum<visa-resource-name>, error out=w1512:errorcluster)  [unwired: 1 out]
          n1228 = VISA Read(VISA resource name=w1513, byte count=u32 1000, error in (no error)=w1512) -> (VISA resource name out=w1510:refnum<visa-resource-name>, read buffer=→"Due read":string, error out=w1511:errorcluster)  [unwired: 1 out]
        }
        n1229 = local read "Command"() -> (w1491:string)
        n1230 = call <vilib>:"Trim Whitespace.vi"("string"=w1491) -> ("trimmed string"=w1490:string)  [unwired: 1 in]
        n1231 = Not Equal?(x=w1490, y="") -> (x != y?=w1497:bool)
        n1232 = case shown="True" w1497 {
          tunnel: w1496 -> [w1515 w1520]
          tunnel: [w1515 w1524] -> w1502
          tunnel: w1495 -> [w1514 w1519]
          tunnel: [w1514 w1522] -> w1501
          tunnel: w1490 -> [_ w1518]
          tunnel: [_ w1521] -> _
          frame False {
            # "DATA  WRITE LOOP"
          }
          frame True {
            n1233 = Concatenate Strings(w1518, "\r\n") -> (w1517:string)
            n1234 = VISA Write(VISA resource name=w1520, write buffer=w1517, error in (no error)=w1519) -> (VISA resource name out=w1524:refnum<visa-resource-name>, return count=w1521:u32, error out=w1523:errorcluster)
            n1235 = flat-sequence {
              tunnel: w1523 -> [w1526]
              tunnel: [w1526] -> w1522
              frame #0 {
                n1236 = local write "Command"("" ("Command")) -> ()
                n1237 = Wait (ms)(milliseconds to wait=u32 5) -> ()  [unwired: 1 out]
              }
            }
          }
        }
        n1238 = VISA Flush I/O Buffer(VISA resource name=w1502) -> (VISA resource name out=w1493:refnum<visa-resource-name>, error out=→"error out 9":errorcluster)  [unwired: 2 in]
      }
      frame Error {
        w1542 = u16 0 items=["None", "XON/XOFF", "RTS/CTS", "XON/XOFF & RTS/CTS", "DTR/DSR", "XON/XOFF & DTR/DSR"] ("flow control (0:none)  2")
        w1540 = u16 10 items=["1.0"=10, "1.5"=15, "2.0"=20] ("stop bits 2")
        w1538 = u16 0 items=["None", "Odd", "Even", "Mark", "Space"] ("parity 2")
        w1539 = u32 10000  # timeout (10sec)
        n1239 = VISA Clear(VISA resource name=w1534, error in (no error)=w1531) -> (VISA resource name out=w1533:refnum<visa-resource-name>, error out=w1532:errorcluster)
        n1240 = VISA Close(VISA resource name=w1533, error in (no error)=w1532) -> (error out=w1535:errorcluster)
        n1241 = call <vilib>:"Clear Errors.vi"("error in (no error)"=w1535) -> ()  [unwired: 5 in, 2 out]
        n1242 = local read "Com Port 2"() -> (w1528:refnum<visa-resource-name>)
        "visa due" <- w1528
        n1243 = call-poly "VISA Configure Serial Port"("VISA resource name"=w1528, "timeout (10sec)"=w1539, "baud rate (9600)"=u32 250000 ("baud rate  2"), "data bits (8)"=u16 8 ("data bits  2"), "parity (0:none)"=w1538, "stop bits (10: 1 bit)"=w1540, "flow control (0:none)"=w1542) -> ("VISA resource name out"=w1543:refnum<visa-resource-name>, "error out"=w1544:errorcluster)  [unwired: 7 in]
        n1244 = flat-sequence {
          tunnel: w1543 -> [w1546]
          tunnel: w1544 -> [w1545]
          tunnel: [w1546] -> w1536
          tunnel: [w1545] -> w1529
          frame #0 {
            n1245 = Wait (ms)(milliseconds to wait=u32 50) -> ()  [unwired: 1 out]
          }
        }
        "Residual Due" <- ""
        "Port 2 Error" <- w1529
      }
    }
    n1246 = local read "Quit"() -> (w1473:bool)
    "Error Due" <- w1478
  }
  n1247 = local write "FRICVALZ"(0.0 ("FRICVALZ")) -> ()
  n1248 = property on="RUN" class="Bool (strict)"("Visible"=TRUE) -> ()  [unwired: 2 in, 2 out]
  n1249 = while {
    tunnel: [w1563] -> _
    tunnel: [w1548] -> w54
    i -> [w1563]
    stop <- w1548 stop-if-true
    n1250 = local read "conststatus"() -> (w1552:dbl)
    n1251 = local read "Main Tab"() -> (w1550:T2)
    n1252 = local read "EDIT"() -> (w1569:bool)
    n1253 = local read "Rate"() -> (w1568:dbl)
    n1254 = case shown="True" w1569 {
      tunnel: [FALSE TRUE] -> w1555
      frame False {
      }
      frame True {
      }
    }
    n1255 = property on="Time slide" class="Slide (strict)"("Scale.Range:Maximum"=2500.0) -> ()  [unwired: 2 in, 2 out]
    n1256 = Equal?(x=w1550, y=T25."About" ("Main Tab")) -> (x = y?=w1561:bool)
    n1257 = Equal?(x=w1552, y=0.0) -> (x = y?=w1553:bool)
    n1258 = Divide(x=1.0, y=w1568) -> (x/y=w1564:dbl)
    "Time 2" <- w1564
    n1259 = case shown="True" w1553 {
      frame False {
      }
      frame True {
        # "C:\\WinDucom\\calibrate WO 2391.dcf"
        n1260 = local write "Lan flag"(22) -> ()
        n1261 = local write "conststatus"(10.0 ("rpm value : 2")) -> ()
        n1262 = String To Path(string="C:\\LAB-IQ\\calibrate WO 2465.dcf") -> (path=w1575:path)
        n1263 = Open/Create/Replace File "Open File"(file path (use dialog)=w1575) -> (refnum out=w1573:refnum<file>)  [unwired: 5 in, 2 out]
        n1264 = for {
          N: 23 -> [_]
          tunnel: w1573 -> [w1584]
          i -> [w1578]
          (unwired) TRUE ("line mode (F)")
